vi "TCPSendResponse.vi"(7 "Quiet":bool, 8 "error in (no error)":errorcluster, 9 "ResponseData":string, 10 "ResponseCode":string="BC", 11 "connection ID":refnum<k5>) -> (0 "error out":errorcluster, 3 "connection ID out":refnum<k5>)   [LabVIEW 2013]
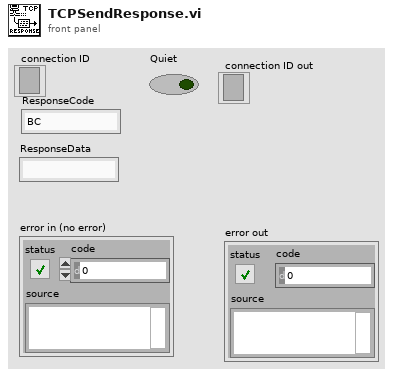
[diagram p1: front panel]
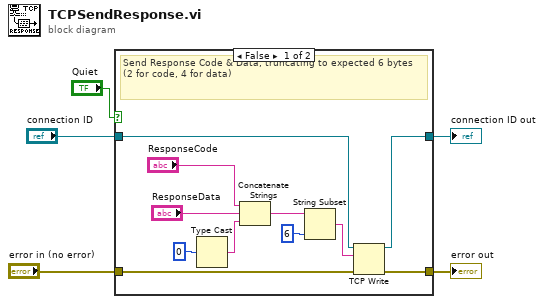
[diagram p0: block diagram]
diagram:
  n1 = case shown="False" "Quiet" {
    tunnel: "connection ID" -> [w16 w18]
    tunnel: [w15 w18] -> w4
    tunnel: "error in (no error)" -> [w14 w17]
    tunnel: [w13 w17] -> w2
    frame False {
      # "Send Response Code & Data, truncating to expected 6 bytes (2 for code, 4 for data)"
      n2 = Type Cast(x=0 ("length (rest)")) -> (*(type *) &x=w9:string)  [unwired: 1 in]
      n3 = Concatenate Strings("ResponseCode", "ResponseData", w9) -> (w11:string)
      n4 = String Subset(string=w11, length (rest)=6 ("length (rest)")) -> (substring=w6:string)  [unwired: 1 in]
      n5 = TCP Write(connection ID=w16, data in=w6, error in (no error)=w14) -> (connection ID out=w15:refnum<k5>, error out=w13:errorcluster)  [unwired: 1 in, 1 out]
    }
    frame True {
      # "QUiet mode, send nothing"
    }
  }
  "error out" <- w2
  "connection ID out" <- w4
